vi "CameraSetTrigger.vi"(8 "error in (no error)":errorcluster, 10 "external?":bool=TRUE, 11 "IMAQdx in":refnum<class "IMAQdx.lvclass">) -> (0 "error out":errorcluster, 2 "attribs":variant[](array[variant]), 3 "IMAQdx out":refnum<class "IMAQdx.lvclass">)   [LabVIEW 2010, in "IMAQdx.lvclass"]
uses:
  <userlib>/BIAS2/classes/IMAQdx/IMAQdx.lvclass
  <userlib>/BIAS2/classes/IMAQdx/IMAQdx.lvclass/IMAQdx.ctl
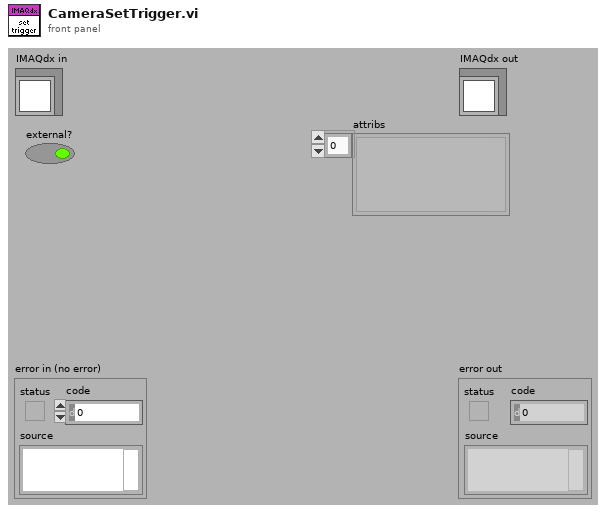
[diagram p1: front panel]
types:
  T1 = typedef "IMAQdx.ctl" = refnum<k21>
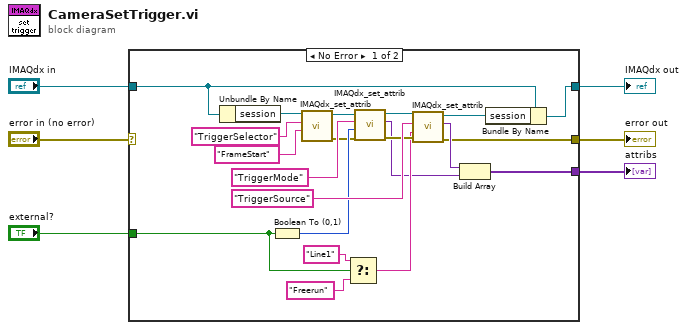
[diagram p0: block diagram]
diagram:
  n1 = case shown="No Error" "error in (no error)" {
    selector: "error in (no error)" -> [_ w29]
    tunnel: [w9 w29] -> w5
    tunnel: [w18 w28] -> w3
    tunnel: "IMAQdx in" -> [w19 w28]
    tunnel: [w8 _] -> w2
    tunnel: "external?" -> [w7 _]
    frame No Error {
      n2 = Unbundle By Name(w19) -> ("session"=w17:refnum<k21>)
      n3 = Boolean To (0,1)(Boolean=w7) -> (0, 1=w23:i16)
      n4 = call <userlib>:"IMAQdx_set_attrib.vi"("value"="FrameStart" ("ActiveAttribute"), "attribute"="TriggerSelector" ("ActiveAttribute"), "IMAQdx in"=w17) -> ("error out"=w13:errorcluster, "IMAQdx out"=w16:T1)  [unwired: 2 in, 1 out]
      n5 = Select(t="Line1", s=w7, f="Freerun") -> (s? t:f=w20:string)
      n6 = call <userlib>:"IMAQdx_set_attrib.vi"("error in"=w13, "value"=w23, "attribute"="TriggerMode" ("ActiveAttribute"), "IMAQdx in"=w16) -> ("error out"=w24:errorcluster, "attrib out"=w10:variant, "IMAQdx out"=w27:T1)  [unwired: 1 in]
      n7 = call <userlib>:"IMAQdx_set_attrib.vi"("error in"=w24, "value"=w20, "attribute"="TriggerSource" ("ActiveAttribute"), "IMAQdx in"=w27) -> ("error out"=w9:errorcluster, "attrib out"=w11:variant, "IMAQdx out"=w12:T1)  [unwired: 1 in]
      n8 = Build Array(w11, w10) -> (w8:variant[])
      n9 = Bundle By Name(cluster=w19, "session"=w12) -> (w18:refnum<class "IMAQdx.lvclass">)
    }
    frame Error {
    }
  }
  "error out" <- w5
  "IMAQdx out" <- w3
  "attribs" <- w2
